vi "Periodic Tasks.vi"(8 "error in":errorcluster) -> ()   [LabVIEW 2014]
doc: "This VI runs in parallel to other tasks. It can contain as many user-defined periodic loops as you need. These can carry out PID or other sorts of timed response."
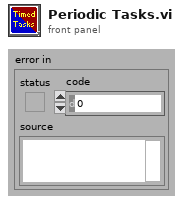
[diagram p1: front panel]
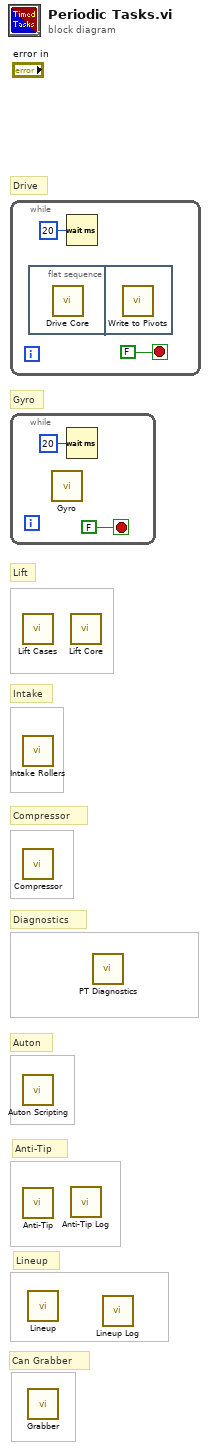
[diagram p0: block diagram]
diagram:
  # "Can Grabber"
  # "Lineup"
  # "Anti-Tip"
  # "Auton"
  # "Drive"
  # "Gyro"
  # "Diagnostics"
  # "Compressor"
  # "Intake"
  # "Lift"
  n1 = while {
    stop <- FALSE stop-if-true
    n2 = flat-sequence {
      frame #0 {
        n3 = call "Drive Core.vi"() -> ()  [unwired: 12 in]
      }
      frame #1 {
        n4 = call "Write to Pivots.vi"() -> ()  [unwired: 12 in]
      }
    }
    n5 = Wait (ms)(milliseconds to wait=u32 20) -> ()  [unwired: 1 out]
  }
  n6 = while {
    stop <- FALSE stop-if-true
    n7 = call "Gyro.vi"() -> ()  [unwired: 12 in]
    n8 = Wait (ms)(milliseconds to wait=u32 20) -> ()  [unwired: 1 out]
  }
  n9 = call "Lift Cases.vi"() -> ()  [unwired: 12 in]
  n10 = call "Intake Rollers.vi"() -> ()  [unwired: 12 in]
  n11 = call "Compressor.vi"() -> ()  [unwired: 12 in]
  n12 = call "Auton Scripting.vi"() -> ()  [unwired: 12 in]
  n13 = call "Anti-Tip.vi"() -> ()  [unwired: 12 in]
  n14 = call "Lineup.vi"() -> ()  [unwired: 12 in]
  n15 = call "Grabber.vi"() -> ()  [unwired: 12 in]
  n16 = call "Lift Core.vi"() -> ()  [unwired: 12 in]
  n17 = call "Anti-Tip Log.vi"() -> ()  [unwired: 12 in]
  n18 = call "PT Diagnostics.vi"() -> ()  [unwired: 12 in]
  n19 = call "Lineup Log.vi"() -> ()  [unwired: 12 in]
